vi "wyswietlInfoOBledzie.vi"(11 "WyjsciaParametry":T1={"Nad. lewo"=FALSE, "Nad.  prawo"=FALSE, "Nad.  gora"=FALSE, "Nad. doł"=FALSE, "Dzialanie"=FALSE, "Pomiar"=FALSE, "Odb. lewo"=FALSE, "Odb.  prawo"=FALSE, "Odb.  gora"=FALSE, "Odb. dol"=FALSE, "Pozostalo punktow"=-1, "Nad. elewacja"=0, "Nad. azymut"=0, "Odb. elewacja"=0, "Odb. azymut"=0, "TCP Error"=FALSE, "TCP Error Code"=0, "LINX Error"=FALSE, "LINX Error Code"=0, "Nastepny elewacja"=0, "Nastepny azymut"=0, "Value Error"=FALSE}) -> (3 "Error info":string)   [LabVIEW 2014]
uses:
  WyjsciaVIs/WyjsciaParametry.ctl
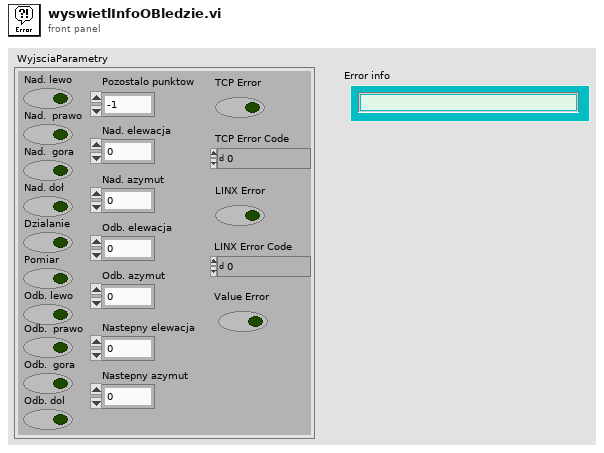
[diagram p1: front panel]
types:
  T1 = typedef "WyjsciaParametry.ctl" = cluster{"Nad. lewo":bool, "Nad.  prawo":bool, "Nad.  gora":bool, "Nad. doł":bool, "Dzialanie":bool, "Pomiar":bool, "Odb. lewo":bool, "Odb.  prawo":bool, "Odb.  gora":bool, "Odb. dol":bool, "Pozostalo punktow":i32, "Nad. elewacja":i32, "Nad. azymut":i32, "Odb. elewacja":i32, "Odb. azymut":i32, "TCP Error":bool, "TCP Error Code":i32, "LINX Error":bool, "LINX Error Code":i32, "Nastepny elewacja":i32, "Nastepny azymut":i32, "Value Error":bool}
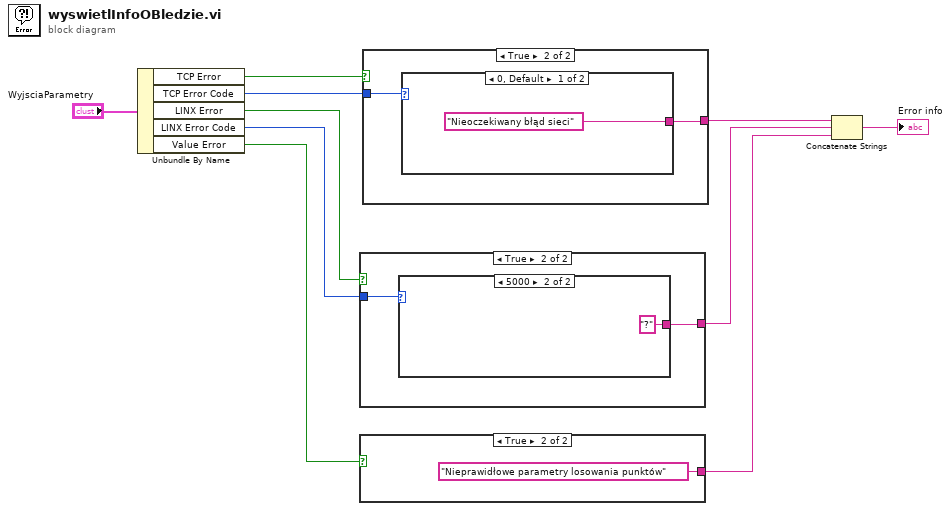
[diagram p0: block diagram]
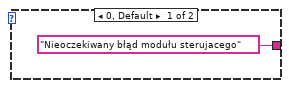
[diagram p4: hidden frame]
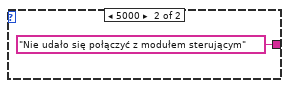
[diagram p6: hidden frame]
diagram:
  n1 = Unbundle By Name("WyjsciaParametry") -> ("TCP Error"=w9:bool, "TCP Error Code"=w8:i32, "LINX Error"=w7:bool, "LINX Error Code"=w6:i32, "Value Error"=w5:bool)
  n2 = case shown="True" w7 {
    tunnel: w6 -> [_ w12]
    tunnel: [_ w11] -> w3
    frame False {
    }
    frame True {
      n3 = case shown="5000" w12 {
        tunnel: ["Nieoczekiwany błąd modułu sterujacego" "?"] -> w11
        frame 0, Default {
        }
        frame 5000 {
        }
      }
    }
  }
  n4 = case shown="True" w5 {
    tunnel: [_ "Nieprawidłowe parametry losowania punktów"] -> w2
    frame False {
    }
    frame True {
    }
  }
  n5 = case shown="True" w9 {
    tunnel: w8 -> [_ w17]
    tunnel: [_ w16] -> w4
    frame False {
    }
    frame True {
      n6 = case shown="0, Default" w17 {
        tunnel: ["Nieoczekiwany błąd sieci" "Nie udało się połączyć z modułem sterującym"] -> w16
        frame 0, Default {
        }
        frame 5000 {
        }
      }
    }
  }
  n7 = Concatenate Strings(w4, w3, w2) -> (→"Error info":string)
